vi "LabVIEW Data Value to Message Element DataType.vi"(8 "error in":errorcluster, 11 "message value":variant) -> (0 "error out":errorcluster, 1 "array":bool, 2 "message name":string, 3 "message element type":T1, 4 "supported":bool)   [LabVIEW 2019, in "grpc-lvsupport.lvlib"]
uses:
  grpc-lvsupport.lvlib
  typeDefs/Message Element Type.ctl
  <vilib>/Utility/Data Type/NI_Data Type.lvlib
  Shared/Well Known Types.ctl
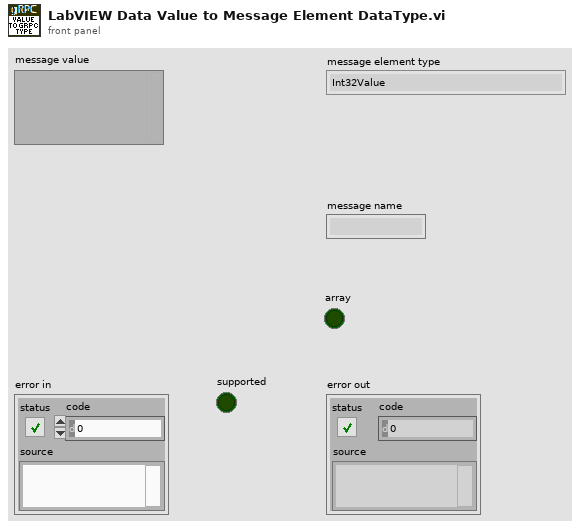
[diagram p1: front panel]
types:
  T1 = typedef "grpc-lvsupport.lvlib/Message Element Type.ctl" = enum32{"Int32Value", "FloatValue", "DoubleValue", "BoolValue", "StringValue", "MessageValue", "Int64Value", "UInt32Value", "UInt64Value", "EnumValue", "Bytes", "Fixed64", "Fixed32", "SFixed64", "SFixed32", "SInt64", "SInt32"}
  T2 = typedef "NI_Data Type.lvlib/Data Type.ctl" = enum8{"Invalid Type", "Void", "I8", "I16", "I32", "I64", "U8", "U16", "U32", "U64", "Single Float", "Double Float", "Extended Float", "Single Complex", "Double Complex", "Extended Complex", "Enum U8", "Enum U16", "Enum U32", "Enum U64", "Single Float With Unit", "Double Float With Unit", "Extended Float With Unit", "Single Complex with Unit", "Double Complex with Unit", "Extended Complex with Unit", "Boolean", "String", "Path", "Picture", "Tag", "Array", "Cluster", "Variant", "LV Variant", "Waveform", "Timestamp", "Digital Waveform", "Digital Data", "ExpressData", "Refnum", "External Data", "VI", "Poly VI", "LabVIEW Class Instance", "Fixed Point", "Set Collection", "Map Collection"}
  T3 = typedef "grpc-lvsupport.lvlib/Well Known Types.ctl" = enum32{"None", "Double2DArray"}
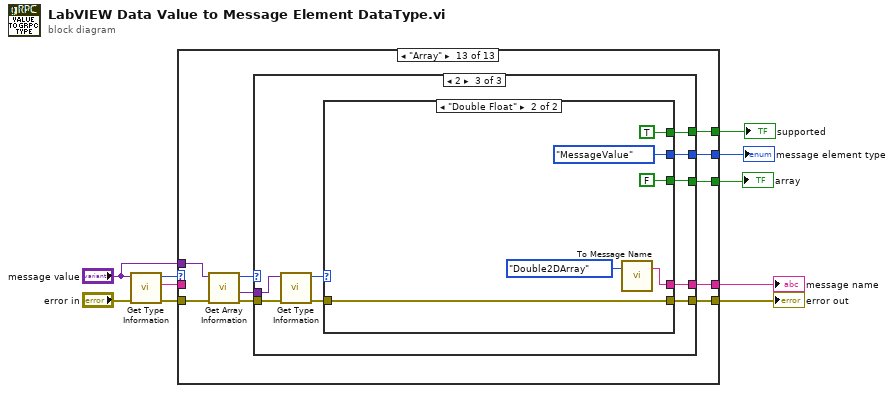
[diagram p0: block diagram]
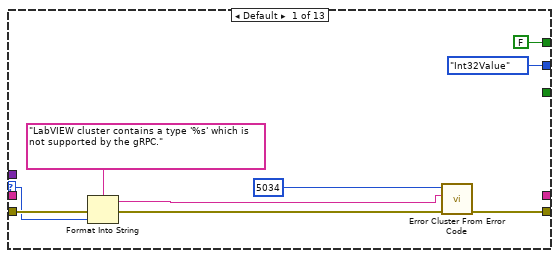
[diagram p2: hidden frame]
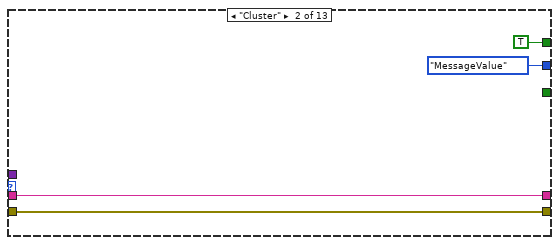
[diagram p3: hidden frame]
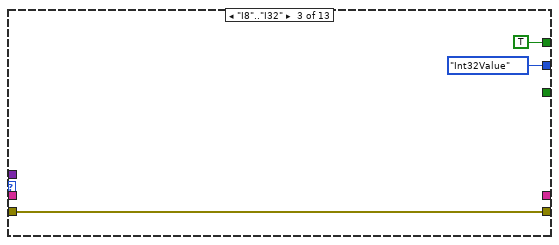
[diagram p4: hidden frame]
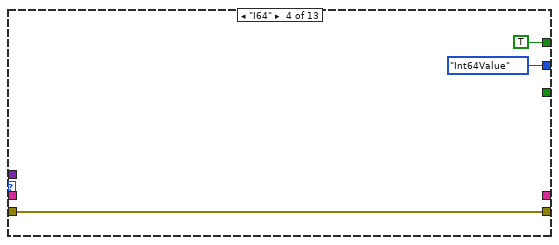
[diagram p5: hidden frame]
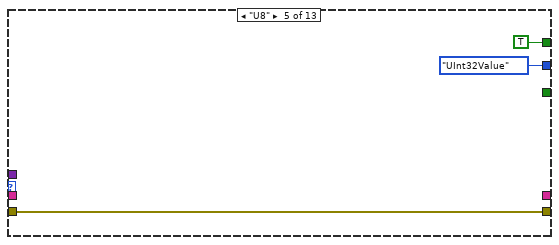
[diagram p6: hidden frame]
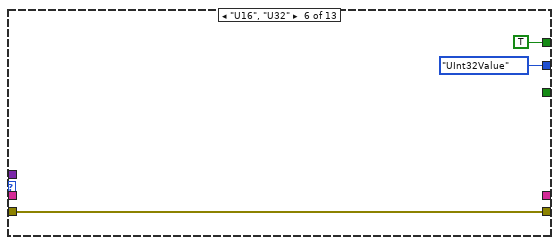
[diagram p7: hidden frame]
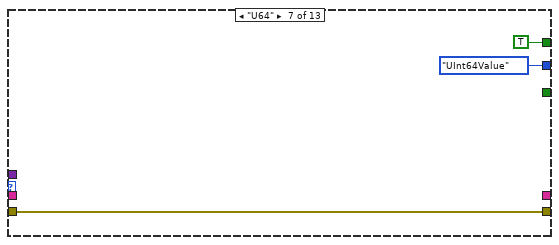
[diagram p8: hidden frame]
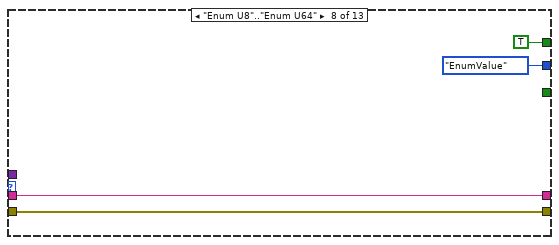
[diagram p9: hidden frame]
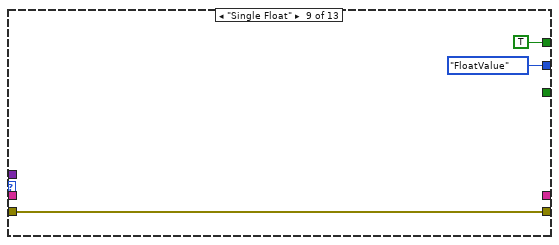
[diagram p10: hidden frame]
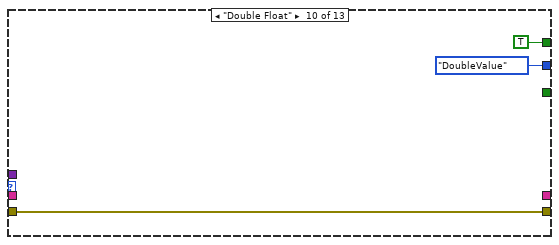
[diagram p11: hidden frame]
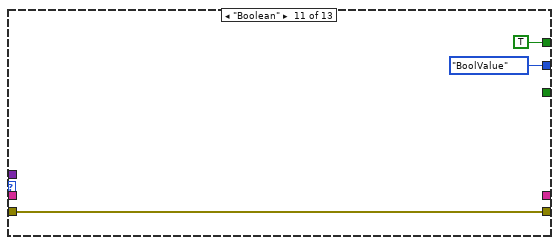
[diagram p12: hidden frame]
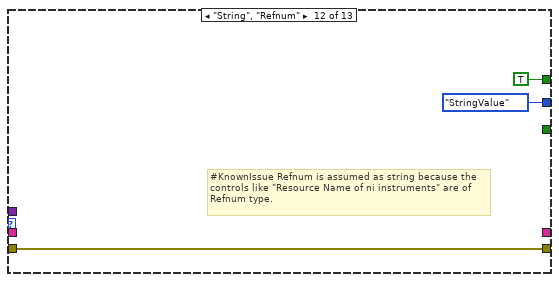
[diagram p13: hidden frame]
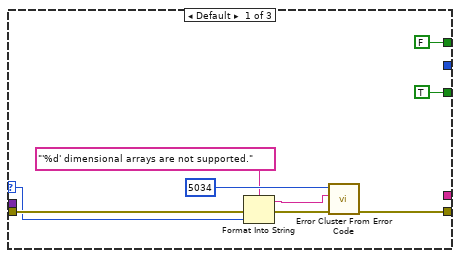
[diagram p14: hidden frame]
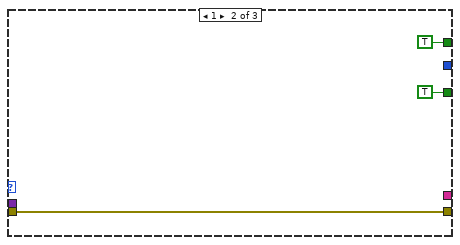
[diagram p15: hidden frame]
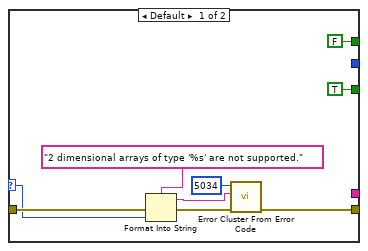
[diagram p16: hidden frame]
diagram:
  n1 = call <vilib>:"Get Type Information.vi"("error in (no error)"="error in", "variant"="message value") -> ("error out"=w5:errorcluster, "name"=w3:string, "type"=w4:T2)  [unwired: 5 in, 2 out]
  n2 = case shown="\"Array\"" w4 {
    selector: w4 -> [w13 _ _ _ _ _ _ _ _ _ _ _ _]
    tunnel: [Message_Element_Type."Int32Value" ("MessageElementType") Message_Element_Type."MessageValue" ("MessageElementType") Message_Element_Type."Int32Value" ("MessageElementType") Message_Element_Type."Int64Value" ("MessageElementType") Message_Element_Type."UInt32Value" ("MessageElementType") Message_Element_Type."UInt32Value" ("MessageElementType") Message_Element_Type."UInt64Value" ("MessageElementType") Message_Element_Type."EnumValue" ("MessageElementType") Message_Element_Type."FloatValue" ("MessageElementType") Message_Element_Type."DoubleValue" ("MessageElementType") Message_Element_Type."BoolValue" ("MessageElementType") Message_Element_Type."StringValue" ("MessageElementType") w56] -> w9
    tunnel: [FALSE TRUE TRUE TRUE TRUE TRUE TRUE TRUE TRUE TRUE TRUE TRUE w64] -> w8
    tunnel: [_ _ _ _ _ _ _ _ _ _ _ _ w63] -> w7
    tunnel: w5 -> [w17 w23 w26 w29 w32 w35 w38 w42 w45 w48 w51 w54 w62]
    tunnel: [w19 w23 w26 w29 w32 w35 w38 w42 w45 w48 w51 w54 w58] -> w10
    tunnel: w3 -> [_ w20 _ _ _ _ _ w39 _ _ _ _ _]
    tunnel: [_ w20 _ _ _ _ _ w39 _ _ _ _ w57] -> w2
    tunnel: "message value" -> [_ _ _ _ _ _ _ _ _ _ _ _ w61]
    frame Default {
      n3 = Format Into String(format string="LabVIEW cluster contains a type '%s' which is not supported by the gRPC.", error in=w17, w13) -> (resulting string=w11:string, error out=w18:errorcluster)  [unwired: 1 in]
      n4 = call <vilib>:"Error Cluster From Error Code.vi"("error in (no error)"=w18, "error message (\"\")"=w11, "error code (0)"=5034) -> ("error out"=w19:errorcluster)  [unwired: 6 in]
    }
    frame "Cluster" {
    }
    frame "I8".."I32" {
    }
    frame "I64" {
    }
    frame "U8" {
    }
    frame "U16", "U32" {
    }
    frame "U64" {
    }
    frame "Enum U8".."Enum U64" {
    }
    frame "Single Float" {
    }
    frame "Double Float" {
    }
    frame "Boolean" {
    }
    frame "String", "Refnum" {
      # "#KnownIssue Refnum is assumed as string because the controls like \"Resource Name of ni instruments\" are of Refnum type."
    }
    frame "Array" {
      n5 = call <vilib>:"Get Array Information.vi"("error in (no error)"=w62, "variant"=w61) -> ("error out"=w59:errorcluster, "array element data type"=w55:variant, "number of dimensions"=w60:i32)  [unwired: 6 in, 1 out]
      n6 = case shown="2" w60 {
        selector: w60 -> [w68 _ _]
        tunnel: [FALSE TRUE w80] -> w64
        tunnel: [TRUE TRUE w79] -> w63
        tunnel: w59 -> [w70 w74 w85]
        tunnel: [w69 w74 w81] -> w58
        tunnel: [_ _ w77] -> w57
        tunnel: [_ _ w78] -> w56
        tunnel: w55 -> [_ _ w84]
        frame Default {
          n7 = Format Into String(format string="'%d' dimensional arrays are not supported.", error in=w70, w68) -> (resulting string=w73:string, error out=w72:errorcluster)  [unwired: 1 in]
          n8 = call <vilib>:"Error Cluster From Error Code.vi"("error in (no error)"=w72, "error message (\"\")"=w73, "error code (0)"=5034) -> ("error out"=w69:errorcluster)  [unwired: 6 in]
        }
        frame 1 {
        }
        frame 2 {
          n9 = call <vilib>:"Get Type Information.vi"("error in (no error)"=w85, "variant"=w84) -> ("error out"=w82:errorcluster, "type"=w83:T2)  [unwired: 5 in, 3 out]
          n10 = case shown="\"Double Float\"" w83 {
            selector: w83 -> [w87 _]
            tunnel: w82 -> [w89 w100]
            tunnel: [w88 w100] -> w81
            tunnel: [FALSE TRUE] -> w80
            tunnel: [TRUE FALSE] -> w79
            tunnel: [_ Message_Element_Type."MessageValue" ("MessageElementType")] -> w78
            tunnel: [_ w95] -> w77
            frame Default {
              n11 = Format Into String(format string="2 dimensional arrays of type '%s' are not supported.", error in=w89, w87) -> (resulting string=w92:string, error out=w91:errorcluster)  [unwired: 1 in]
              n12 = call <vilib>:"Error Cluster From Error Code.vi"("error in (no error)"=w91, "error message (\"\")"=w92, "error code (0)"=5034) -> ("error out"=w88:errorcluster)  [unwired: 6 in]
            }
            frame "Double Float" {
              n13 = call "To Message Name.vi"("well known type"=Well_Known_Types."Double2DArray") -> ("message name"=w95:string)  [unwired: 1 in, 1 out]
            }
          }
        }
      }
    }
  }
  "message element type" <- w9
  "supported" <- w8
  "array" <- w7
  "error out" <- w10
  "message name" <- w2
